vi "Gray Morphological Reconstruction H-Dome.vi"() -> ()   [LabVIEW 2014]
doc: "This example demonstrates a grayscale morphological reconstruction as part of a H-Dome process. First, a specified value is subtracted from the source image. Next, a morphological reconstruction is applied using the subtracted image as a marker. The resulting image is subtracted from the source to get the H-Dome. A set of points are overlayed on the source to show the position of H-Domes in the original image."
uses:
  <vilib>/vision/NI_Vision_Development_Module.lvlib
panel:
  in  "Images":T1(tab)=enum."Overlay Result"
  out "Source Image":T2(plugin-control)
  out "Image Marker":T2(plugin-control)
  out "Morphological Reconstruction":T2(plugin-control)
  out "Isolated Particles":T2(plugin-control)
  out "Result Image":T2(plugin-control)
  # "Overview: Demonstrate the use of the Gray Morphological Reconstruction feature of Vision Development Module.\nRequirements: Vision Development Module.\nInstructions:\n1. Run the VI.\n2. Navigate the tabs to view the intermediate images."
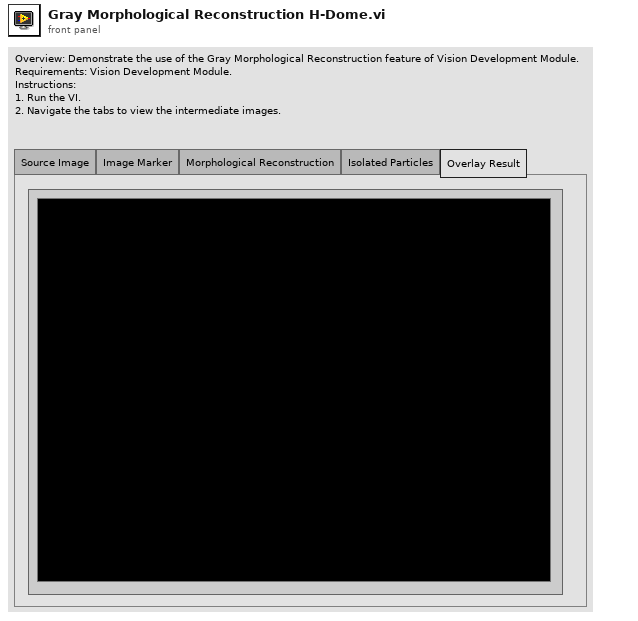
[diagram p1: front panel]
types:
  T1 = enum32{"Source Image", "Image Marker", "Morphological Reconstruction", "Isolated Particles", "Overlay Result"}
  T2 = typedef "IMAQ Image.ctl" = refnum<image>
  T3 = cluster{"Area":dbl, "Number of Holes":dbl, "Bounding Rect":cluster{"Left":dbl, "Top":dbl, "Right":dbl, "Bottom":dbl}, "Center of Mass":cluster{"X":dbl, "Y":dbl}, "Orientation":dbl, "Dimensions":cluster{"Width":dbl, "Height":dbl}}[]
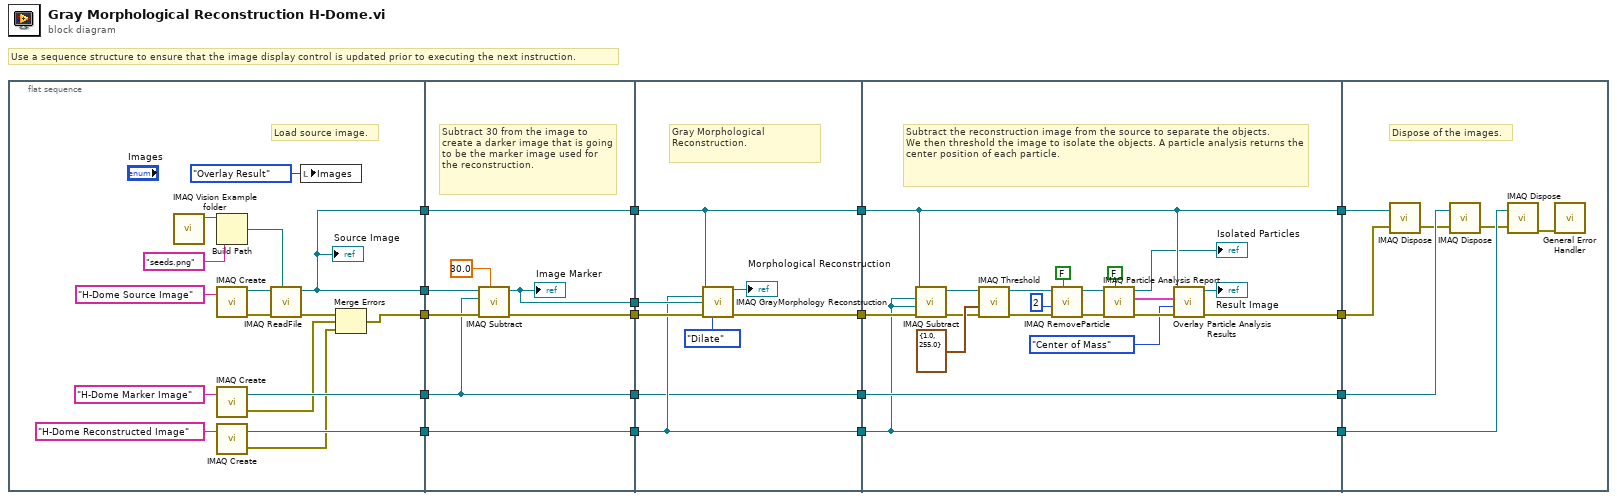
[diagram p0: block diagram]
diagram:
  # "Use a sequence structure to ensure that the image display control is updated prior to executing the next instruction."
  n1 = flat-sequence {
    tunnel: [w24] -> w18
    tunnel: [w28] -> w17
    tunnel: [w24] -> w15
    tunnel: [w26] -> w12
    tunnel: [w20] -> w5
    tunnel: w18 -> [w41]
    tunnel: w17 -> [w35]
    tunnel: [w42] -> w16
    tunnel: w15 -> [w42]
    tunnel: [w39] -> w14
    tunnel: [w37] -> w13
    tunnel: w12 -> [w37]
    tunnel: [w36] -> w11
    tunnel: [w35] -> w8
    tunnel: w5 -> [w40]
    tunnel: [w50] -> w4
    tunnel: w16 -> [w50]
    tunnel: w14 -> [w48]
    tunnel: w13 -> [w45]
    tunnel: w11 -> [w49]
    tunnel: [w46] -> w3
    tunnel: [w45] -> w2
    tunnel: [w44] -> w1
    tunnel: w8 -> [w44]
    tunnel: w4 -> [w52]
    tunnel: w3 -> [w70]
    tunnel: w2 -> [w59]
    tunnel: [w52] -> w10
    tunnel: [w55] -> w9
    tunnel: w1 -> [w60]
    tunnel: [w60] -> w7
    tunnel: [w59] -> w6
    tunnel: w10 -> [w77]
    tunnel: w9 -> [w76]
    tunnel: w7 -> [w75]
    tunnel: w6 -> [w74]
    frame #0 {
      # "Load source image."
      n2 = call "IMAQ Vision Example folder.vi"() -> ("Example Image Path"=w32:path)  [unwired: 11 in]
      n3 = Build Path(base path=w32, name or relative path="seeds.png") -> (appended path=w25:path)
      n4 = call "IMAQ Create"("Image Name"="H-Dome Source Image") -> ("New Image"=w31:T2, "error out"=w30:errorcluster)  [unwired: 3 in, 1 out]
      n5 = call "IMAQ Create"("Image Name"="H-Dome Marker Image") -> ("New Image"=w28:T2, "error out"=w22:errorcluster)  [unwired: 3 in, 1 out]
      n6 = call "IMAQ Create"("Image Name"="H-Dome Reconstructed Image") -> ("New Image"=w26:T2, "error out"=w21:errorcluster)  [unwired: 3 in, 1 out]
      n7 = call "IMAQ ReadFile"("File Path"=w25, "error in (no error)"=w30, "Image"=w31) -> ("error out"=w23:errorcluster, "Image Out"=w24:T2)  [unwired: 2 in, 5 out]
      "Source Image" <- w24
      n8 = local write "Images"(T1."Overlay Result" ("Images")) -> ()
      n9 = Merge Errors(w23, w22, w21) -> (w20:errorcluster)
    }
    frame #1 {
      # "Subtract 30 from the image to create a darker image that is going to be the marker image used for the reconstruction."
      n10 = call "IMAQ Subtract"("Image Src A"=w41, "Constant"=sgl 30.0 ("Value"), "Image Dst"=w35, "error in (no error)"=w40) -> ("Image Dst Out"=w36:T2, "error out"=w39:errorcluster)  [unwired: 1 in, 2 out]
      "Image Marker" <- w36
    }
    frame #2 {
      # "Gray Morphological Reconstruction."
      n11 = call "IMAQ GrayMorphology Reconstruction"("Image Src"=w50, "Image Dst"=w45, "Image Marker"=w49, "error in (no error)"=w48, "Operation"=enum32{"Dilate", "Erode"}."Dilate") -> ("Image Dst Out"=→"Morphological Reconstruction":T2, "error out"=w46:errorcluster)  [unwired: 3 in, 6 out]
    }
    frame #3 {
      # "Subtract the reconstruction image from the source to separate the objects.\nWe then threshold the image to isolate the objects. A particle analysis returns the center position of each particle."
      n12 = call "IMAQ Subtract"("Image Src A"=w52, "Image Dst"=w59, "Image Src B"=w59, "error in (no error)"=w70) -> ("Image Dst Out"=w66:T2, "error out"=w65:errorcluster)  [unwired: 1 in, 2 out]
      n13 = call "IMAQ Threshold"("error in (no error)"=w65, "Range"=cluster{"Lower value":sgl, "Upper value":sgl} {"Lower value"=1.0, "Upper value"=255.0}, "Image Src"=w66) -> ("error out"=w64:errorcluster, "Image Dst Out"=w53:T2)  [unwired: 3 in, 4 out]
      n14 = call "IMAQ RemoveParticle"("Square/Hexa (Square)"=FALSE, "error in (no error)"=w64, "Number of Erosion"=2, "Image Src"=w53) -> ("error out"=w61:errorcluster, "Image Dst Out"=w68:T2)  [unwired: 3 in, 3 out]
      n15 = call "IMAQ Particle Analysis Report"("Connectivity 4/8 (8)"=FALSE, "error in (no error)"=w61, "Image"=w68) -> ("error out"=w58:errorcluster, "Particle Reports (Pixels)"=w57:T3, "Image Out (duplicate)"=→"Isolated Particles":T2)  [unwired: 6 out]
      n16 = call "Overlay Particle Analysis Results.vi"("error in"=w58, "Overlay"=enum16{"Bounding Box", "Center of Mass"}."Center of Mass", "Particle Reports (Pixels)"=w57, "Image"=w52) -> ("error out"=w55:errorcluster, "Image Out"=→"Result Image":T2)  [unwired: 6 in]
    }
    frame #4 {
      # "Dispose of the images."
      n17 = call "IMAQ Dispose"("Image"=w77, "error in (no error)"=w76) -> ("error out"=w73:errorcluster)  [unwired: 1 in, 3 out]
      n18 = call "IMAQ Dispose"("Image"=w75, "error in (no error)"=w73) -> ("error out"=w72:errorcluster)  [unwired: 1 in, 3 out]
      n19 = call "IMAQ Dispose"("Image"=w74, "error in (no error)"=w72) -> ("error out"=w71:errorcluster)  [unwired: 1 in, 3 out]
      n20 = call <vilib>:"General Error Handler.vi"("error in (no error)"=w71) -> ()  [unwired: 10 in, 5 out]
    }
  }
